vi "ClearGraphData.vi"(8 "error in (no error)":errorcluster caption="entrée d'erreur (pas d'erreur)", 10 "GraphNumber":i32, 11 "Interface en entrée":refnum<class "Interface.lvclass"> caption="DNL_LabVIEW Object in") -> (0 "error out":errorcluster caption="sortie d'erreur", 2 "OldGraphIndex":i32, 3 "Interface en sortie":refnum<class "Interface.lvclass"> caption="DNL_LabVIEW Object out")   [LabVIEW 2019, in "Interface.lvclass"]
uses:
  Interface.lvclass
  Interface.lvclass/Interface.ctl
  CurveSetup.ctl
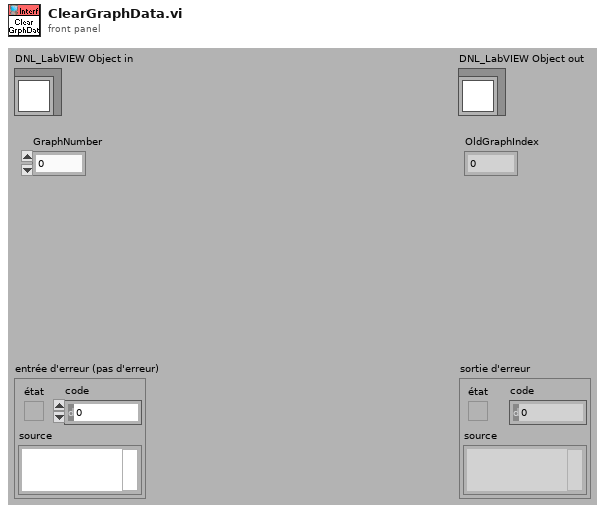
[diagram p1: front panel]
types:
  T1 = typedef "Interface.lvclass/CurveSetup.ctl" = cluster{"CurveName":string, "YParam":string, "XParam":string, "ZParam ":string, "GroupName":string, "LinWdth":u8, "PntCol":u32, "LinCol":u32, "LablFor":u8, "XScale":u32, "YScale":u32, "Interpol":u8, "DisplayName":string, "FillType":i16, "LineStyle":u8, "PntStyle":u8, "BarTyp":u8, "GraphIndex":i32, "Visible":bool, "XScaleName":string, "YScaleName":string, "XYGraph_Ref":refnum<vi>, "Data Only":bool, "DataQ Ref":refnum<queue>, "XParQ Ref":refnum<queue>, "XParamInd":i32, "ScanInd":i32}
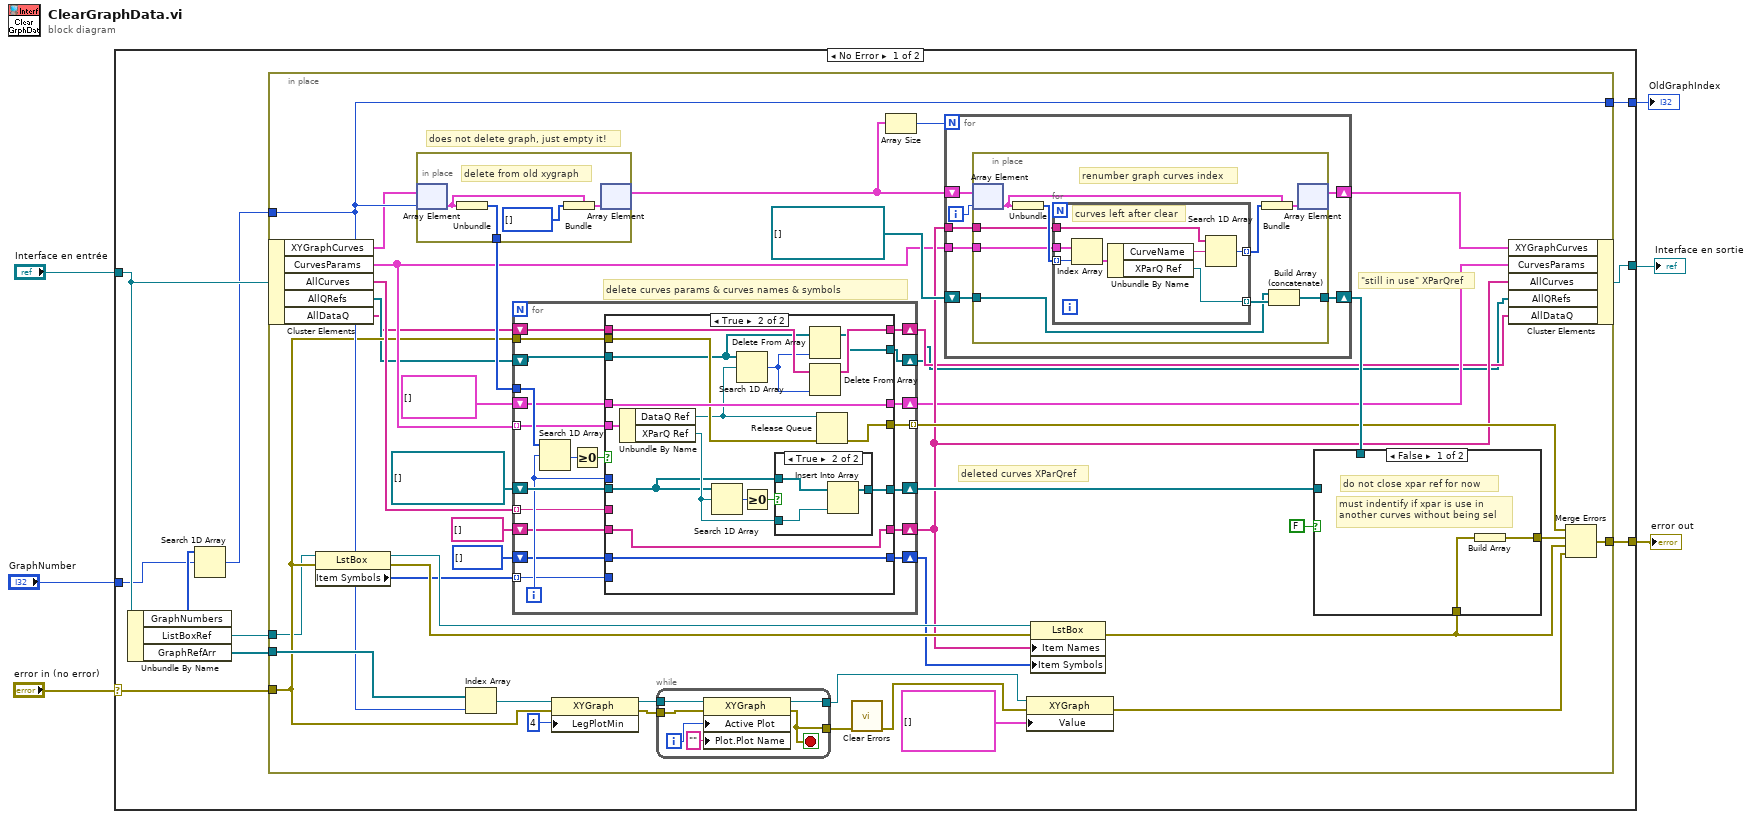
[diagram p0: block diagram]
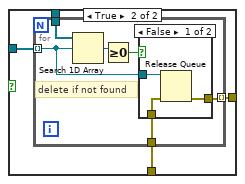
[diagram p2: hidden frame]
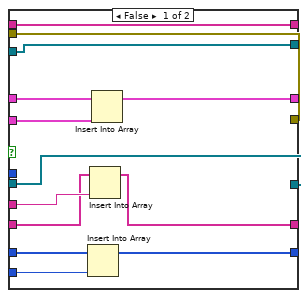
[diagram p4: hidden frame]
diagram:
  n1 = case shown="No Error" "error in (no error)" {
    selector: "error in (no error)" -> [w16 w164]
    tunnel: [w11 w164] -> w5
    tunnel: [w15 w163] -> w3
    tunnel: "Interface en entrée" -> [w14 w163]
    tunnel: "GraphNumber" -> [w8 _]
    tunnel: [w13 _] -> w1
    frame No Error {
      n2 = Unbundle By Name(w14) -> ("GraphNumbers"=w9:i32[], "ListBoxRef"=w10:refnum<vi>, "GraphRefArr"=w12:refnum<vi>[])
      n3 = Search 1D Array(1D array=w9, element=w8) -> (index of element=w7:i32)  [unwired: 1 in]
      n4 = in-place {
        in-place-border: w7 -> [w46]
        in-place-border: w16 -> [w26]
        in-place-border: [w46] -> w13
        in-place-border: w12 -> [w58]
        in-place-border: [w49] -> w11
        in-place-border: w10 -> [w23]
        # "does not delete graph, just empty it!"
        # "deleted curves XParQref"
        # "\"still in use\" XParQref"
        # "delete curves params & curves names & symbols"
        n5 = in-place-cluster #1(w14) -> ("XYGraphCurves"=w28:cluster{"Tableau":i32[]}[], "CurvesParams"=w29:T1[], "AllCurves"=w37:string[], "AllQRefs"=w21:refnum<queue>[], "AllDataQ"=w20:string[])
        n6 = property on="Nœud de propriété" class="LstBox"(reference=w23, error in=w26) -> (reference out=w50:refnum<vi>, error out=w48:errorcluster, "Item Symbols"=w36:i32[])
        n7 = in-place {
          in-place-border: [w160] -> w53
          # "delete from old xygraph"
          n8 = in-place-array #2(w28, w46) -> (w162:cluster{"Tableau":i32[]})
          n9 = Unbundle(w162) -> ("Tableau"=w160:i32[])
          n10 = Bundle(cluster=w162, "Tableau"=i32[] []) -> (w161:cluster{"Tableau":i32[]})
          n11 = in-place-array #2(w161) -> (w27:cluster{"Tableau":i32[]}[])  [unwired: 1 out]
        }
        n12 = Index Array(array=w58, index=w46) -> (element=w56:refnum<vi>)
        n13 = for {
          tunnel: w53 -> [w114]
          tunnel: [w118] -> w42 mode=indexing
          tunnel: w26 -> [w117]
          shift-right: [w115] -> w47
          shift-left: refnum<queue>[] [] -> [w116]
          tunnel: w29 -> [w111] mode=indexing
          shift-right: [w110] -> w32
          shift-left: T1[] [] -> [w109]
          tunnel: w37 -> [w107] mode=indexing
          tunnel: w36 -> [w106] mode=indexing
          shift-right: [w105] -> w33
          shift-left: string[] [] -> [w104]
          shift-right: [w103] -> w30
          shift-left: i32[] [] -> [w102]
          shift-right: [w99] -> w19
          shift-left: w20 -> [w100]
          shift-right: [w98] -> w18
          shift-left: w21 -> [w101]
          i -> [w108]
          n14 = Search 1D Array(1D array=w114, element=w108) -> (index of element=w112:i32)  [unwired: 1 in]
          n15 = Greater Or Equal To 0?(x=w112) -> (x >= 0?=w113:bool)
          n16 = case shown="True" w113 {
            tunnel: [w121 w148] -> w118
            tunnel: w117 -> [w121 w139]
            tunnel: w116 -> [w122 w144]
            tunnel: [w122 w143] -> w115
            tunnel: w111 -> [w131 w140]
            tunnel: [w130 w142] -> w110
            tunnel: w109 -> [w129 w142]
            tunnel: w108 -> [_ _]
            tunnel: w107 -> [w128 _]
            tunnel: w106 -> [w125 _]
            tunnel: [w127 w138] -> w105
            tunnel: w104 -> [w126 w138]
            tunnel: [w124 w141] -> w103
            tunnel: w102 -> [w123 w141]
            tunnel: w101 -> [w119 w134]
            tunnel: w100 -> [w120 w136]
            tunnel: [w120 w135] -> w99
            tunnel: [w119 w132] -> w98
            frame False {
              n17 = Insert Into Array(array=w123, new element=w125) -> (w124:i32[])  [unwired: 1 in]
              n18 = Insert Into Array(array=w126, new element=w128) -> (w127:string[])  [unwired: 1 in]
              n19 = Insert Into Array(array=w129, new element=w131) -> (w130:T1[])  [unwired: 1 in]
            }
            frame True {
              n20 = Unbundle By Name(w140) -> ("DataQ Ref"=w137:refnum<queue>, "XParQ Ref"=w145:refnum<queue>)
              n21 = Search 1D Array(1D array=w144, element=w145) -> (index of element=w147:i32)  [unwired: 1 in]
              n22 = Search 1D Array(1D array=w134, element=w137) -> (index of element=w133:i32)  [unwired: 1 in]
              n23 = Greater Or Equal To 0?(x=w147) -> (x >= 0?=w146:bool)
              n24 = case shown="True" w146 {
                tunnel: w145 -> [_ w150]
                tunnel: w144 -> [w149 w152]
                tunnel: [w149 w151] -> w143
                frame False {
                }
                frame True {
                  n25 = Insert Into Array(array=w152, new element=w150) -> (w151:refnum<queue>[])  [unwired: 1 in]
                }
              }
              n26 = Delete From Array(array=w134, index=w133) -> (array with subset deleted=w132:refnum<queue>[])  [unwired: 1 in, 1 out]
              n27 = Delete From Array(array=w136, index=w133) -> (array with subset deleted=w135:string[])  [unwired: 1 in, 1 out]
              n28 = Release Queue(queue=w137, error in (no error)=w139) -> (error out=w148:errorcluster)  [unwired: 1 in, 2 out]
            }
          }
        }
        n29 = property class="XYGraph"(reference=w56, error in=w26, "LegPlotMin"=u32 4 ("Légende : minimum de tracés")) -> (reference out=w24:refnum<vi>, error out=w55:errorcluster)
        n30 = while {
          tunnel: w24 -> [w158]
          tunnel: w55 -> [w156]
          tunnel: [w154] -> w54
          tunnel: [w153] -> w39
          i -> [w155]
          stop <- w154 stop-if-true
          n31 = property class="XYGraph"(reference=w158, error in=w156, "Active Plot"=w155, "Plot.Plot Name"="" ("Tracé.Nom du tracé")) -> (reference out=w153:refnum<vi>, error out=w154:errorcluster)
        }
        n32 = call <vilib>:"Clear Errors.vi"("error in (no error)"=w54) -> ("error out"=w38:errorcluster)  [unwired: 5 in, 1 out]
        n33 = Array Size(array=w27) -> (size(s)=w52:i32)
        n34 = for {
          N: w52 -> [_]
          shift-right: [w77] -> w51
          shift-left: w27 -> [w81]
          tunnel: w29 -> [w79]
          tunnel: w33 -> [w78]
          shift-right: [w76] -> w43
          shift-left: refnum<queue>[] [] -> [w75]
          i -> [w80]
          n35 = in-place {
            in-place-border: w79 -> [w89]
            in-place-border: w78 -> [w88]
            in-place-border: [w83] -> w76
            in-place-border: w75 -> [w82]
            # "renumber graph curves index"
            n36 = in-place-array #3(w81, w80) -> (w87:cluster{"Tableau":i32[]})
            n37 = Unbundle(w87) -> ("Tableau"=w90:i32[])
            n38 = for {
              tunnel: w90 -> [w97] mode=indexing
              tunnel: w89 -> [w96]
              tunnel: w88 -> [w93]
              tunnel: [w92] -> w85 mode=indexing
              tunnel: [w91] -> w84 mode=indexing
              # "curves left after clear"
              n39 = Index Array(array=w96, index=w97) -> (element=w95:T1)
              n40 = Unbundle By Name(w95) -> ("CurveName"=w94:string, "XParQ Ref"=w91:refnum<queue>)
              n41 = Search 1D Array(1D array=w93, element=w94) -> (index of element=w92:i32)  [unwired: 1 in]
            }
            n42 = Bundle(cluster=w87, "Tableau"=w85) -> (w86:cluster{"Tableau":i32[]})
            n43 = Build Array (concatenate)(w82, w84) -> (w83:refnum<queue>[])
            n44 = in-place-array #3(w86) -> (w77:cluster{"Tableau":i32[]}[])  [unwired: 1 out]
          }
        }
        n45 = property class="XYGraph"(reference=w39, error in=w38, "Value"=cluster{dbl[], dbl[]}[] []) -> (error out=w22:errorcluster)  [unwired: 1 out]
        n46 = property class="LstBox"(reference=w50, error in=w48, "Item Names"=w33, "Item Symbols"=w30) -> (error out=w25:errorcluster)  [unwired: 1 out]
        n47 = case shown="False" FALSE {
          tunnel: w47 -> [_ w64]
          tunnel: w43 -> [_ w63]
          tunnel: [w59 w62] -> w41
          tunnel: w25 -> [w60 w61]
          frame False {
            # "must indentify if xpar is use in\nanother curves without being sel"
            # "do not close xpar ref for now"
            n48 = Build Array(w60) -> (w59:errorcluster[])
          }
          frame True {
            n49 = for {
              tunnel: w64 -> [w67] mode=indexing
              tunnel: w63 -> [w70]
              tunnel: w61 -> [w66]
              tunnel: [w65] -> w62 mode=indexing
              # "delete if not found"
              n50 = Search 1D Array(1D array=w70, element=w67) -> (index of element=w69:i32)  [unwired: 1 in]
              n51 = Greater Or Equal To 0?(x=w69) -> (x >= 0?=w68:bool)
              n52 = case shown="False" w68 {
                tunnel: w67 -> [w73 _]
                tunnel: w66 -> [w72 w74]
                tunnel: [w71 w74] -> w65
                frame False {
                  n53 = Release Queue(queue=w73, error in (no error)=w72) -> (error out=w71:errorcluster)  [unwired: 1 in, 2 out]
                }
                frame True {
                }
              }
            }
          }
        }
        n54 = in-place-cluster #1("XYGraphCurves"=w51, "CurvesParams"=w32, "AllCurves"=w33, "AllQRefs"=w18, "AllDataQ"=w19) -> (w15:refnum<class "Interface.lvclass">)
        n55 = Merge Errors(w42, w41, w25, w22) -> (w49:errorcluster)
      }
    }
    frame Error {
    }
  }
  "error out" <- w5
  "Interface en sortie" <- w3
  "OldGraphIndex" <- w1
